vi "Target Motor Current Magnitude Limiter.vi"(11 "Motor Command":dbl) -> (3 "Motor Command Out":dbl)   [LabVIEW 2018]
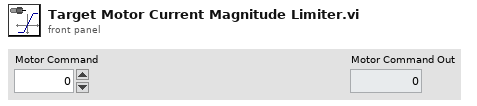
[diagram p1: front panel]
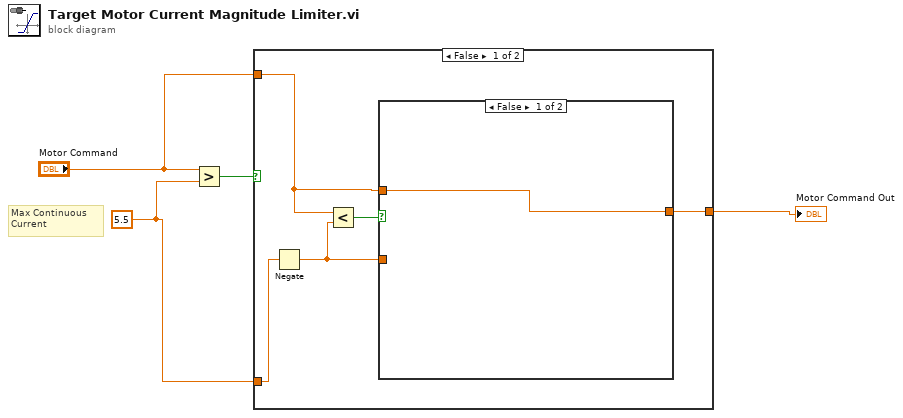
[diagram p0: block diagram]
diagram:
  w3 = 5.5
  # "Max Continuous \nCurrent"
  n1 = Greater?(x="Motor Command", y=w3) -> (0:w4:bool)
  n2 = case shown="False" w4 {
    tunnel: w3 -> [w6 w12]
    tunnel: [w8 w12] -> w2
    tunnel: "Motor Command" -> [w7 _]
    frame False {
      n3 = Negate(x=w6) -> (-x=w5:dbl)
      n4 = Less?(x=w7, y=w5) -> (x < y?=w9:bool)
      n5 = case shown="False" w9 {
        tunnel: [w10 w11] -> w8
        tunnel: w7 -> [w10 _]
        tunnel: w5 -> [_ w11]
        frame False {
        }
        frame True {
        }
      }
    }
    frame True {
    }
  }
  "Motor Command Out" <- w2
